vi "Funcion_LEER_B.vi"(9 "PIPES ENTRADA":cluster{"PIPE_IN":i32, "PIPE_OUT":i32}, 11 "error in (no error)":errorcluster) -> (0 "subarray":bool[](array[boolean]), 1 "PIPES SALIDA":cluster{"PIPE_IN":i32, "PIPE_OUT":i32}, 3 "error out":errorcluster)   [LabVIEW 2016]
uses:
  microchip_solutions_v2013-06-15/USB/Tools/MCHPUSB Custom Driver/Mpusbapi/Dll/Borland_C/mpusbapi.dll
panel:
  out "plength*":i32
  out "pData*":i32
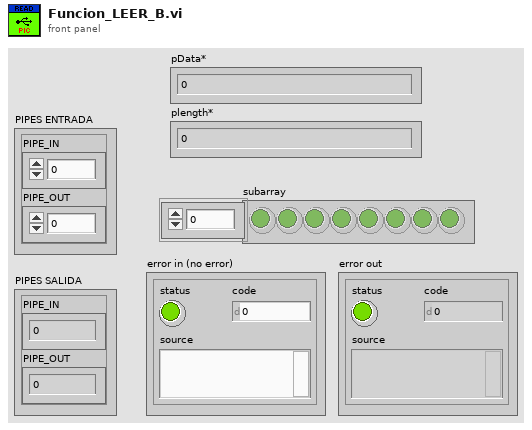
[diagram p1: front panel]
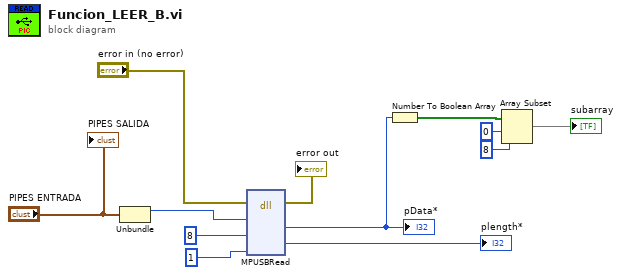
[diagram p0: block diagram]
diagram:
  n1 = Unbundle("PIPES ENTRADA") -> ("PIPE_IN"=w3:i32)  [unwired: 1 out]
  n2 = dll-call lib="C:/microchip_solutions_v2013-06-15/USB/Tools/MCHPUSB Custom Driver/Mpusbapi/Dll/Borland_C/mpusbapi.dll" fn="MPUSBRead"(error in="error in (no error)", "PIPE IN"=w3, "dwlen"=8, "dwMilliseconds"=1) -> (error out=→"error out":errorcluster, "pData*"=w6:i32, "plength"=→"plength*":i32)  [unwired: 8 in, 1 out]
  "pData*" <- w6
  n3 = Number To Boolean Array(number=w6) -> (Boolean array=w7:bool[])
  n4 = Array Subset(array=w7, index=0, length=8) -> (→"subarray":bool[])
  "PIPES SALIDA" <- "PIPES ENTRADA"
